vi "PID Drive.vi"(0 "Setpoint Distance":dbl, 1 "PID gains":T1={"proportional gain (Kc)"=0.8, "integral time (Ti, min)"=0.0, "derivative time (Td, min)"=0.001}, 5 "Setpoint Angle":dbl, 7 "Speed":dbl, 9 "Reset Encoder":bool, 11 "Reset Gyro":bool) -> (4 "Encoder Distance":dbl, 6 "Gyro Angle":dbl)   [LabVIEW 2015]
uses:
  <vilib>/Rock Robotics/WPI/Utilities/WPI_GetSetVariantRefNum.vi
  <vilib>/addons/control/pid/pid.llb/PID Structure Conversion (DBL).vi
  <vilib>/addons/control/pid/pid.llb/PID Control Input Filter (DBL).vi
  <vilib>/addons/control/pid/pid.llb/PID (DBL).vi
  <vilib>/addons/control/pid/NI_PID_pid.lvlib
panel:
  out "Turning Output":dbl(knob) scale=-0.5..0.5
  out "Driving Output":dbl(knob) scale=-0.5..0.5
  out "At Distance":bool
  out "Error Graph":dbl(graph)
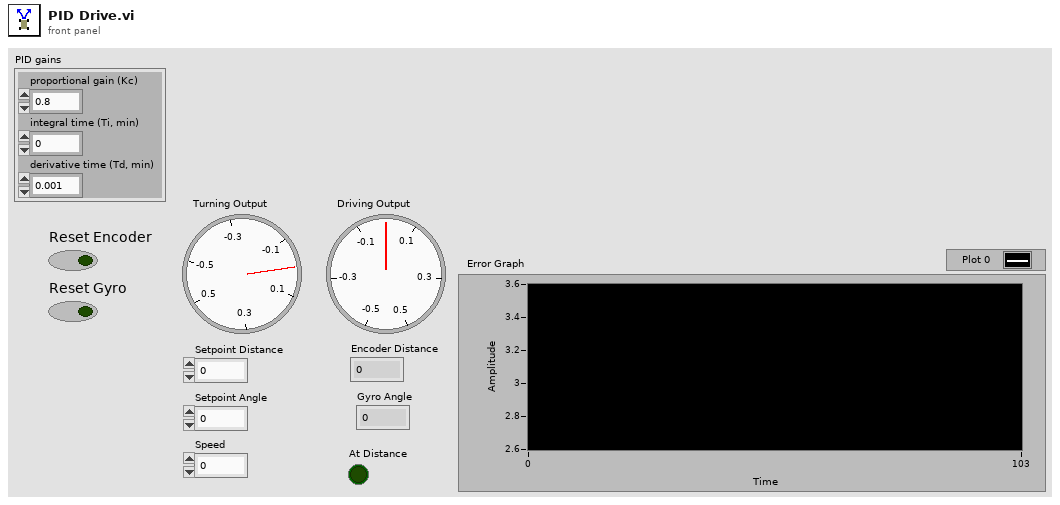
[diagram p1: front panel]
types:
  T1 = cluster{"proportional gain (Kc)":dbl, "integral time (Ti, min)":dbl, "derivative time (Td, min)":dbl}
  T2 = typedef "WPI_GyroDevRef.ctl" = cluster{"DevStatus":errorcluster, "Analog Channel":T3, "Offset":dbl, "Gain (VoltsPerDegree/Second)":dbl, "Gyro Type":enum16{"Analog", "XRS450"}, "Handle":i32, "SPI Bus":T4, "Device Found":bool, "Sample Rate":dbl, "Calibrate On Open":bool}
  T3 = typedef "FPGA_AIChannel.ctl" = enum8{"AI 0", "AI 1", "AI 2", "AI 3", "AI MXP 0", "AI MXP 1", "AI MXP 2", "AI MXP 3", "Invalid"}
  T4 = typedef "spi_bus.ctl" = enum16{"SPI On-Board, CS0", "SPI On-Board, CS1", "SPI On-Board, CS2", "SPI On-Board, CS3", "SPI MXP", "Invalid"}
  T5 = typedef "WPI_EncoderDevRef.ctl" = cluster{"DevStatus":errorcluster, "EncoderIndex":T6, "CounterIndex":T7, "DistancePerCount":dbl, "Decoding Type":T8}
  T6 = typedef "FPGA_EncoderIdx.ctl" = enum8{"Enc 0", "Enc 1", "Enc 2", "Enc 3", "Enc 4", "Enc 5", "Enc 6", "Enc 7", "Invalid"}
  T7 = typedef "FPGA_CounterCtrSystemIndex.ctl" = enum8{"Ctr 0", "Ctr 1", "Ctr 2", "Ctr 3", "Ctr 4", "Ctr 5", "Ctr 6", "Ctr 7", "Invalid"}
  T8 = typedef "WPI_EncoderType.ctl" = enum16{"1x", "2x", "4x"}
  T9 = typedef "WPI_RobotDriveDevRef.ctl" = cluster{"DevStatus":errorcluster, "Motors[]":T10[], "Square Inputs":bool, "Max Output":dbl}
  T10 = typedef "WPI_MotorControlDeviceRef.ctl" = cluster{"DeviceStatus":errorcluster, "Type":T11, "PWM":cluster{"PWM Channel":T12, "DeadBand":T13}, "CAN":cluster{"Device Number":u8, "Control Mode":T14, "Semaphore":T15, "Max Vout":dbl, "TalonSRX Control Mode":T16}, "Invert":bool}
  T11 = typedef "WPI_MotorControlType.ctl" = enum16{"PWM", "CAN", "CANTalonSRX"}
  T12 = typedef "FPGA_DIOPWMChannel.ctl" = enum8{"PWM 0", "PWM 1", "PWM 2", "PWM 3", "PWM 4", "PWM 5", "PWM 6", "PWM 7", "PWM 8", "PWM 9", "PWM MXP 0", "PWM MXP 1", "PWM MXP 2", "PWM MXP 3", "PWM MXP 4", "PWM MXP 5", "PWM MXP 6", "PWM MXP 7", "PWM MXP 8", "PWM MXP 9", "Invalid"}
  T13 = typedef "WPI_PWMDeadband.ctl" = cluster{"Name":string, "maxPositivePwm":i32, "minPositivePwm":i32, "centerPwm":i32, "maxNegativePwm":i32, "minNegativePwm":i32, "angularRange":u16}
  T14 = typedef "WPI_CANJaguar_ControlMode.ctl" = enum8{"Percent VBus", "Current", "Speed", "Position", "Voltage"}
  T15 = typedef "Semaphore RefNum" = refnum<k1>
  T16 = typedef "WPI_CANTalonSRX_APIControlMode.ctl" = enum8{"Percent VBus", "Speed", "Position", "Slave", "Unchanged / Invalid", "Voltage Compensation", "Current", "Motion Profile"}
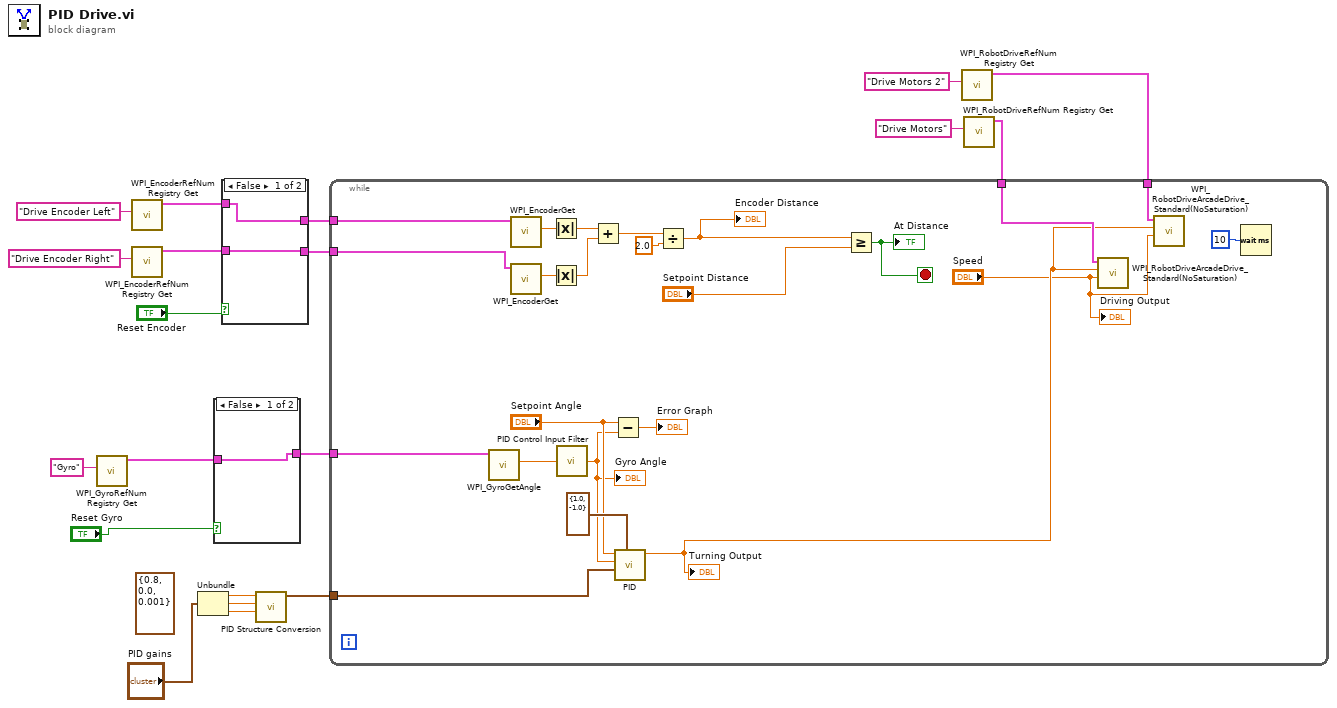
[diagram p0: block diagram]
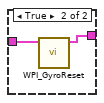
[diagram p2: hidden frame]
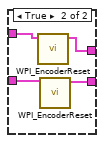
[diagram p3: hidden frame]
diagram:
  (unwired) T1 {"proportional gain (Kc)"=0.8, "integral time (Ti, min)"=0.0, "derivative time (Td, min)"=0.001} ("PID gains")
  n1 = call <vilib>:"WPI_GyroRefNum Registry Get.vi"("refnum name"="Gyro") -> ("GyroDevRef"=w11:T2)  [unwired: 9 in, 1 out]
  n2 = call <vilib>:"WPI_EncoderRefNum Registry Get.vi"("refnum name"="Drive Encoder Left") -> ("EncoderDevRef"=w17:T5)  [unwired: 9 in, 1 out]
  n3 = call <vilib>:"WPI_EncoderRefNum Registry Get.vi"("refnum name"="Drive Encoder Right") -> ("EncoderDevRef"=w18:T5)  [unwired: 9 in, 1 out]
  n4 = Unbundle("PID gains") -> ("proportional gain (Kc)"=w9:dbl, "integral time (Ti, min)"=w8:dbl, "derivative time (Td, min)"=w7:dbl)
  n5 = case shown="False" "Reset Gyro" {
    tunnel: w11 -> [w21 w23]
    tunnel: [w21 w22] -> w10
    frame False {
    }
    frame True {
      n6 = call <vilib>:"WPI_GyroReset.vi"("GyroDevRef"=w23) -> ("GyroDevRef"=w22:T2)  [unwired: 9 in, 1 out]
    }
  }
  n7 = case shown="False" "Reset Encoder" {
    tunnel: w18 -> [w24 w29]
    tunnel: w17 -> [w25 w28]
    tunnel: [w25 w27] -> w16
    tunnel: [w24 w26] -> w15
    frame False {
    }
    frame True {
      n8 = call <vilib>:"WPI_EncoderReset.vi"("EncoderDevRef"=w28) -> ("EncoderDevRef"=w27:T5)  [unwired: 9 in, 1 out]
      n9 = call <vilib>:"WPI_EncoderReset.vi"("EncoderDevRef"=w29) -> ("EncoderDevRef"=w26:T5)  [unwired: 9 in, 1 out]
    }
  }
  n10 = call-poly <vilib>:"PID Structure Conversion.vi"("derivative"=w7, "integral"=w8, "proportional"=w9) -> ("PID gains"=w6:T1)  [unwired: 8 in]
  n11 = call <vilib>:"WPI_RobotDriveRefNum Registry Get.vi"("refnum name"="Drive Motors 2") -> ("RobotDriveDevRef"=w2:T9)  [unwired: 1 in, 9 out]
  n12 = call <vilib>:"WPI_RobotDriveRefNum Registry Get.vi"("refnum name"="Drive Motors") -> ("RobotDriveDevRef"=w4:T9)  [unwired: 1 in, 9 out]
  n13 = while {
    tunnel: w16 -> [w37]
    tunnel: w15 -> [w36]
    tunnel: w10 -> [w35]
    tunnel: w6 -> [w34]
    tunnel: w4 -> [w33]
    tunnel: w2 -> [w32]
    stop <- w38 stop-if-true
    n14 = call <vilib>:"WPI_GyroGetAngle.vi"("GyroDevRef"=w35) -> ("Angle"=w50:dbl)  [unwired: 6 in, 4 out]
    n15 = call <vilib>:"WPI_EncoderGet.vi"("EncoderDevRef"=w37) -> ("Distance"=w45:dbl)  [unwired: 5 in, 5 out]
    n16 = call <vilib>:"WPI_EncoderGet.vi"("EncoderDevRef"=w36) -> ("Distance"=w46:dbl)  [unwired: 5 in, 5 out]
    n17 = Absolute Value(x=w45) -> (abs(x)=w44:dbl)
    n18 = Absolute Value(x=w46) -> (abs(x)=w43:dbl)
    n19 = call-poly <vilib>:"PID Control Input Filter.vi"("input"=w50) -> ("output"=w40:dbl)  [unwired: 4 in]
    "Gyro Angle" <- w40
    n20 = Add(x=w44, y=w43) -> (x+y=w48:dbl)
    n21 = Subtract(x="Setpoint Angle", y=w40) -> (x-y=→"Error Graph":dbl)
    n22 = call-poly <vilib>:"PID.vi"("output range"=cluster{"output high":dbl, "output low":dbl} {"output high"=1.0, "output low"=-1.0}, "PID gains"=w34, "process variable"=w40, "setpoint"="Setpoint Angle") -> ("output"=w31:dbl)  [unwired: 6 in, 1 out]
    "Turning Output" <- w31
    n23 = Divide(x=w48, y=2.0) -> (x/y=w49:dbl)
    "Encoder Distance" <- w49
    n24 = Greater Or Equal?(x=w49, y="Setpoint Distance") -> (x >= y?=w38:bool)
    "At Distance" <- w38
    n25 = call <vilib>:"WPI_RobotDriveArcadeDrive_Standard(NoSaturation).vi"("Y axis value"="Speed", "X axis value"=w31, "RobotDriveDevRef"=w33) -> ()  [unwired: 1 in, 8 out]
    n26 = call <vilib>:"WPI_RobotDriveArcadeDrive_Standard(NoSaturation).vi"("Y axis value"="Speed", "X axis value"=w31, "RobotDriveDevRef"=w32) -> ()  [unwired: 1 in, 8 out]
    n27 = Wait (ms)(milliseconds to wait=u32 10) -> ()  [unwired: 1 out]
    "Driving Output" <- "Speed"
  }
